vi "_003.vi"() -> ()   [LabVIEW 2024]
panel:
  out "1/x":dbl
  in  "x":dbl
  out "-x":dbl
  in  "x":dbl
  out "x^2":dbl
  in  "x":dbl
  out "sqrt(x)":dbl
  in  "x":dbl
  out "ceil(x): smallest int >= x":dbl
  in  "x":dbl
  out "floor(x): largest int <= x":dbl
  in  "x":dbl
  out "nearest integer value":dbl
  in  "x":dbl
  out "abs(x)":dbl
  in  "x":dbl
  out "product":dbl
  in  "numeric array 2":dbl[](array[numeric])
  out "sum":dbl
  in  "numeric array":dbl[](array[numeric])
  out "x-1":dbl
  in  "x":dbl
  out "x+1":dbl
  in  "x":dbl
  # "Numeric Symbols :"
  # "(Basics)"
  # "Increment :"
  # "Decrement :"
  # "Add array elements :"
  # "Multiple array elements :"
  # "Absolute value :"
  # "Round to nearest :"
  # "Round towards +infinity :"
  # "Round towards -infinity :"
  # "Square root :"
  # "Square :"
  # "Neagative :"
  # "Reciprocal :"
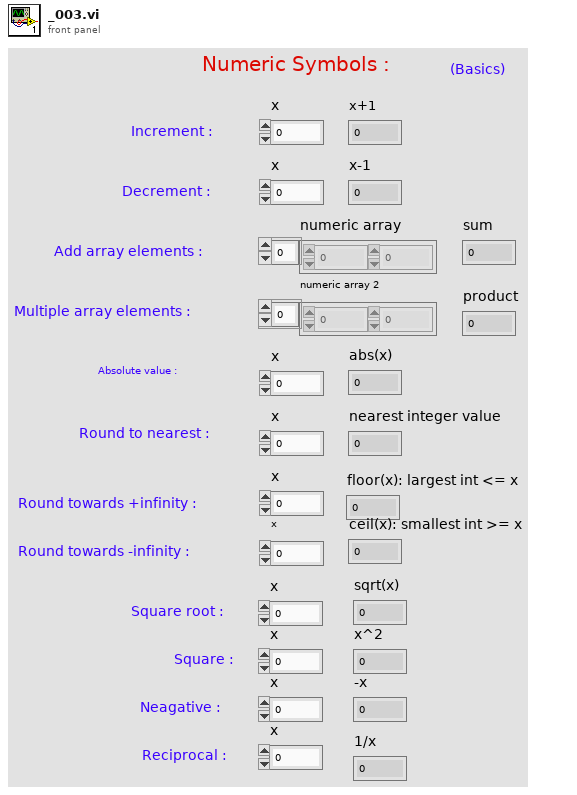
[diagram p1: front panel]
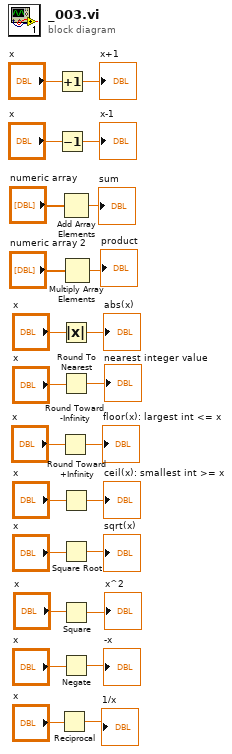
[diagram p0: block diagram]
diagram:
  n1 = Increment(x="x") -> (x+1=→"x+1":dbl)
  n2 = Decrement(x="x") -> (x-1=→"x-1":dbl)
  n3 = Reciprocal(x="x") -> (1/x=→"1/x":dbl)
  n4 = Round Toward -Infinity(1:"x") -> (0:→"floor(x): largest int <= x":dbl)
  n5 = Add Array Elements(numeric array="numeric array") -> (sum=→"sum":dbl)
  n6 = Absolute Value(x="x") -> (abs(x)=→"abs(x)":dbl)
  n7 = Round To Nearest(number="x") -> (nearest integer value=→"nearest integer value":dbl)
  n8 = Round Toward +Infinity(x="x") -> (ceil(x): smallest int >= x=→"ceil(x): smallest int >= x":dbl)
  n9 = Square Root(x="x") -> (sqrt(x)=→"sqrt(x)":dbl)
  n10 = Square(x="x") -> (x^2=→"x^2":dbl)
  n11 = Negate(x="x") -> (-x=→"-x":dbl)
  n12 = Multiply Array Elements(1:"numeric array 2") -> (0:→"product":dbl)
